vi "Dequeue Broadcast Message.vi"(8 "error in (no error)":errorcluster, 9 "Timeout (-1)":i32=-1, 11 "Event Registration Refnum":refnum<event-registration>) -> (0 "error out":errorcluster, 1 "Message Data":variant, 2 "Message":string, 3 "Event Registration Refnum Out":refnum<event-registration>, 4 "Timed Out?":bool, 5 "Sender":string)   [LabVIEW 2020, in "Broadcast Event Helpers.lvlib"]
doc: "Dequeues the next incomming broadcast message.\n\nThis VI is deperecated and a 1:1 replacement is available in the support directory. The event helper methods will be removed from TF.lvlib in a future release and should be replaced with the support library."
uses:
  Broadcast Event Helpers.lvlib
  Process/Protected/Broadcasting/Broadcast Message Cluster.ctl
  Process/Process.lvclass
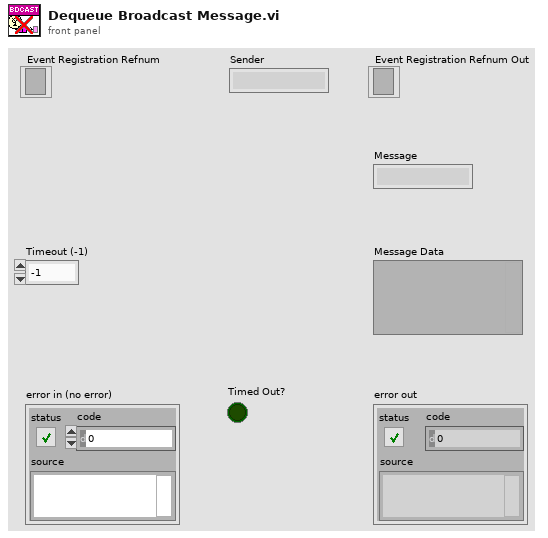
[diagram p1: front panel]
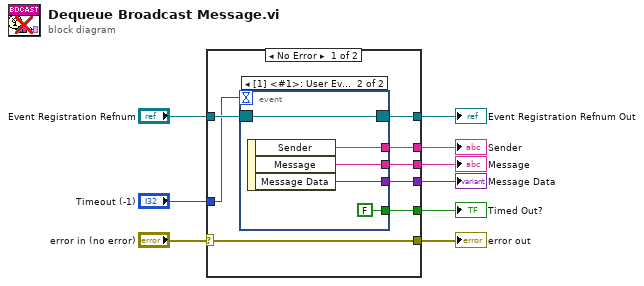
[diagram p0: block diagram]
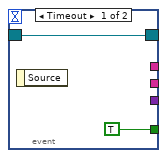
[diagram p2: hidden frame]
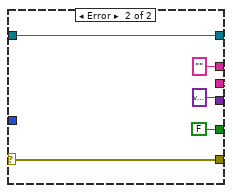
[diagram p3: hidden frame]
diagram:
  n1 = case shown="No Error" "error in (no error)" {
    selector: "error in (no error)" -> [w10 w30]
    tunnel: "Event Registration Refnum" -> [w17 w25]
    tunnel: "Timeout (-1)" -> [w16 _]
    tunnel: [w15 w25] -> w7
    tunnel: [w14 "" ("Sender")] -> w6
    tunnel: [w13 "" ("Message")] -> w5
    tunnel: [w12 variant ("Message Data")] -> w4
    tunnel: [w11 FALSE] -> w3
    tunnel: [w10 w30] -> w1
    frame No Error {
      n2 = event shown="[1] <#1>: User Event" {
        selector: w17 -> [w19 w21]
        dyn-events: [w19 w21] -> w15
        timeout: w16 -> [_ _]
        tunnel: [_ w24] -> w14
        tunnel: [_ w23] -> w13
        tunnel: [_ w22] -> w12
        tunnel: [TRUE FALSE] -> w11
        event Timeout {
          n3 = event-data() -> ()  [unwired: 1 in, 1 out]
        }
        event User Event {
          n4 = event-data() -> ("Sender"=w24:string, "Message"=w23:string, "Message Data"=w22:variant)  [unwired: 1 in]
        }
      }
    }
    frame Error {
    }
  }
  "Event Registration Refnum Out" <- w7
  "Message Data" <- w4
  "Message" <- w5
  "Sender" <- w6
  "error out" <- w1
  "Timed Out?" <- w3
